vi "Celsius_Fahrenheit_converter.vi"(0 "C":dbl) -> (1 "F":dbl, 2 "alarm":bool)   [LabVIEW 2022 SP3]
doc: "Celsius to Fahrnheit converter"
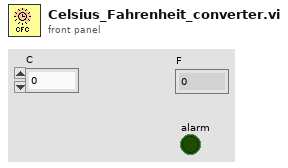
[diagram p1: front panel]
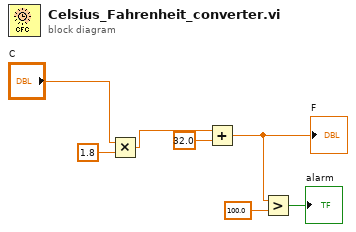
[diagram p0: block diagram]
diagram:
  n1 = Multiply(x="C", y=1.8) -> (x*y=w5:dbl)
  n2 = Add(x=w5, y=32.0) -> (x+y=w3:dbl)
  "F" <- w3
  n3 = Greater?(x=w3, y=100.0) -> (0:→"alarm":bool)
